vi "AES-Cipher-text.vi"(5 "Initializer Vector":u8[](array[numeric]), 7 "Operation Mode":T1, 8 "error in (no error)":errorcluster, 10 "Cipher Key":u8[](array[numeric]), 11 "Message in":u8[](array[numeric])) -> (0 "error out":errorcluster, 3 "Ciphered message":u8[](array[numeric]))   [LabVIEW 2011, in "i3-external-encryption.lvlib"]
doc: "Encripts the <b>text</b> in using the cipher and the given <b>Operation Mode</b> using AES algorithm.\nThe cipher key and initialization vector should be a hex-string (ASCII values 0-f).\n\nCAUTION:\nThis VI is not secure, it does not protect the memory of the encryption, key and unencrypted data.\n\n(c) Ton Plomp, 2011\nTHIS SOFTWARE IS PROVIDED AS IS, AND ANY WARRANTY IS REJECTED"
uses:
  i3-external-encryption.lvlib
  AES-Modes.ctl
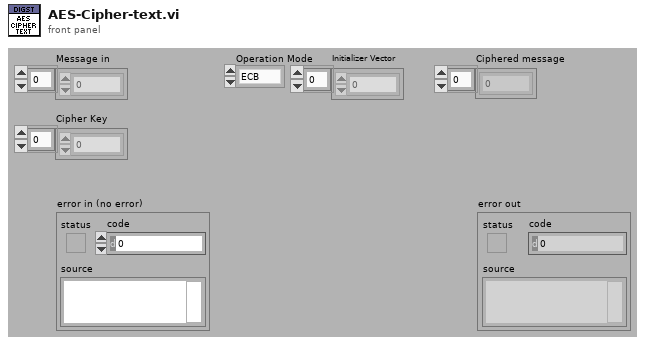
[diagram p1: front panel]
types:
  T1 = typedef "i3-external-encryption.lvlib/AES-Modes.ctl" = enum16{"ECB", "CBC", "CFB128", "OFB"}
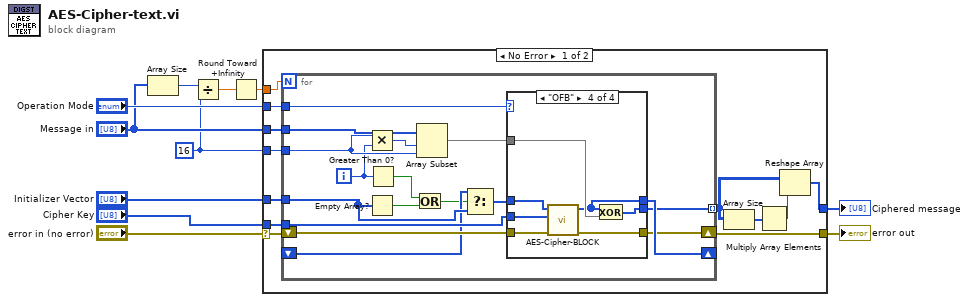
[diagram p0: block diagram]
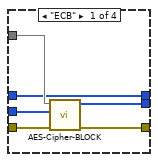
[diagram p2: hidden frame]
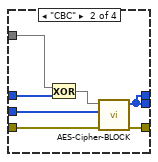
[diagram p3: hidden frame]
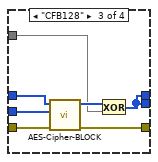
[diagram p4: hidden frame]
diagram:
  w4 = 16 ("y")
  n1 = Array Size(array="Message in") -> (size(s)=w5:i32)
  n2 = Divide(x=w5, y=w4) -> (x/y=w7:dbl)
  n3 = Round Toward +Infinity(x=w7) -> (ceil(x): smallest int >= x=w6:dbl)
  n4 = case shown="No Error" "error in (no error)" {
    selector: "error in (no error)" -> [w19 w68]
    tunnel: "Message in" -> [w23 _]
    tunnel: [w18 w68] -> w11
    tunnel: "Cipher Key" -> [w22 _]
    tunnel: w6 -> [w21 _]
    tunnel: w4 -> [w20 _]
    tunnel: [w12 _] -> w10
    tunnel: "Operation Mode" -> [w17 _]
    tunnel: "Initializer Vector" -> [w16 _]
    frame No Error {
      n5 = for {
        N: w21 -> [_]
        tunnel: w23 -> [w34]
        tunnel: w22 -> [w40]
        tunnel: w20 -> [w38]
        shift-right: [w26] -> w18
        shift-left: w19 -> [w37]
        tunnel: w17 -> [w36]
        shift-right: [w35] -> _
        shift-left: _ -> [w31]
        tunnel: w16 -> [w33]
        tunnel: [w24] -> w14 mode=indexing
        i -> [w29]
        n6 = Multiply(x=w38, y=w29) -> (x*y=w39:i32)
        n7 = Empty Array?(array=w33) -> (empty?=w28:bool)
        n8 = Greater Than 0?(x=w29) -> (x > 0?=w30:bool)
        n9 = Or(x=w30, y=w28) -> (x .or. y?=w27:bool)
        n10 = Array Subset(array=w34, index=w39, length=w38) -> (w25:u8[])
        n11 = Select(t=w31, s=w27, f=w33) -> (s? t:f=w32:u8[])
        n12 = case shown="\"OFB\"" w36 {
          tunnel: w40 -> [w46 w53 w60 w67]
          tunnel: w25 -> [w45 w47 w55 w63]
          tunnel: w37 -> [w44 w52 w59 w66]
          tunnel: [w43 w49 w54 w62] -> w24
          tunnel: [w42 w51 w58 w65] -> w26
          tunnel: w32 -> [w41 w50 w57 w64]
          tunnel: [w41 w49 w54 w61] -> w35
          frame "ECB" {
            n13 = call "AES-Cipher-BLOCK.vi"("error in (no error)"=w44, "Cipher Key"=w46, "Plain [U8]"=w45) -> ("error out"=w42:errorcluster, "cipher [U8]"=w43:u8[])  [unwired: 7 in]
          }
          frame "CBC" {
            n14 = Exclusive Or(1:w50, 2:w47) -> (0:w48:u8[])
            n15 = call "AES-Cipher-BLOCK.vi"("error in (no error)"=w52, "Cipher Key"=w53, "Plain [U8]"=w48) -> ("error out"=w51:errorcluster, "cipher [U8]"=w49:u8[])  [unwired: 7 in]
          }
          frame "CFB128" {
            n16 = call "AES-Cipher-BLOCK.vi"("error in (no error)"=w59, "Cipher Key"=w60, "Plain [U8]"=w57) -> ("error out"=w58:errorcluster, "cipher [U8]"=w56:u8[])  [unwired: 7 in]
            n17 = Exclusive Or(1:w55, 2:w56) -> (0:w54:u8[])
          }
          frame "OFB" {
            n18 = call "AES-Cipher-BLOCK.vi"("error in (no error)"=w66, "Cipher Key"=w67, "Plain [U8]"=w64) -> ("error out"=w65:errorcluster, "cipher [U8]"=w61:u8[])  [unwired: 7 in]
            n19 = Exclusive Or(1:w63, 2:w61) -> (0:w62:u8[])
          }
        }
      }
      n20 = Array Size(array=w14) -> (size(s)=w15:i32[])
      n21 = Multiply Array Elements(1:w15) -> (0:w13:i32)
      n22 = Reshape Array(w14, w13) -> (w12:u8[])
    }
    frame Error {
    }
  }
  "error out" <- w11
  "Ciphered message" <- w10
